vi "Sim Signal 1 CH.vi"(8 "Voltage 2":dbl, 9 "Filter 2":enum16{"Highpass", "Lowpass"}(ring), 10 "Filter 1":enum16{"Highpass", "Lowpass"}(ring), 11 "Voltage 1":dbl) -> (3 "Signal 1 Out":dbl)   [LabVIEW 2010]
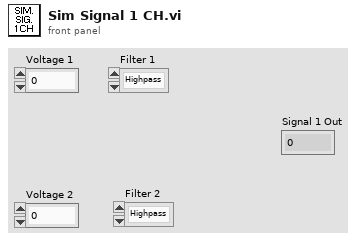
[diagram p1: front panel]
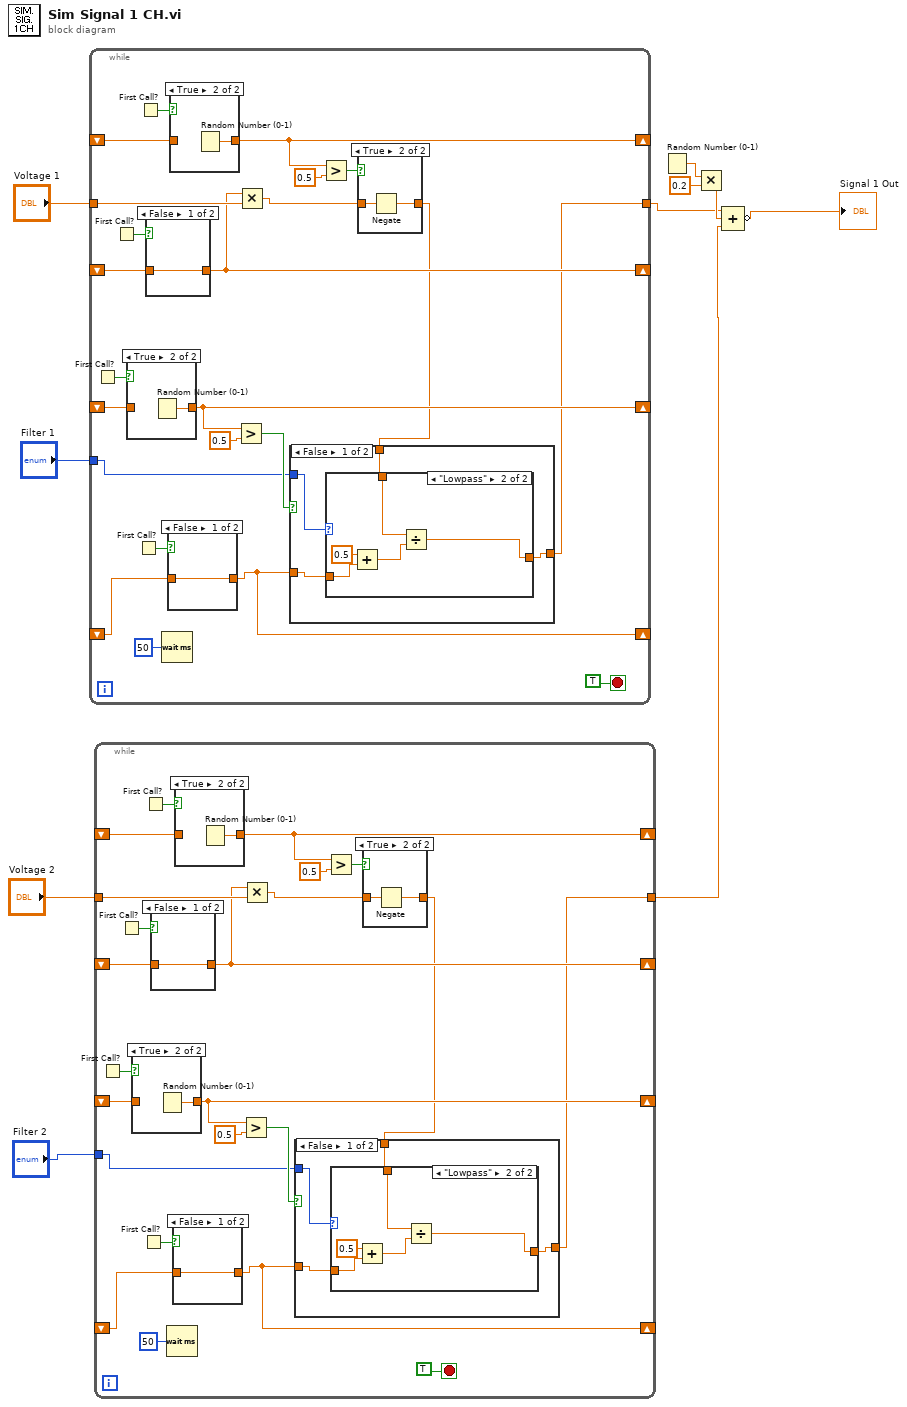
[diagram p0: block diagram]
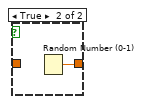
[diagram p2: hidden frame]
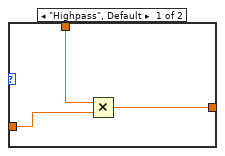
[diagram p3: hidden frame]
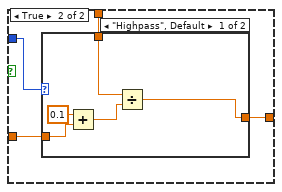
[diagram p4: hidden frame]
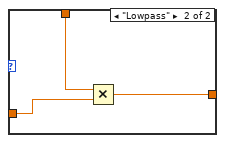
[diagram p5: hidden frame]
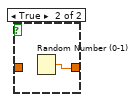
[diagram p9: hidden frame]
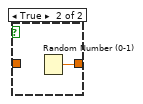
[diagram p10: hidden frame]
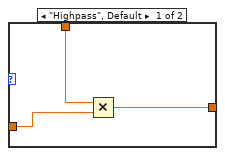
[diagram p11: hidden frame]
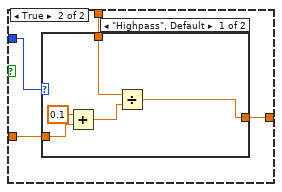
[diagram p12: hidden frame]
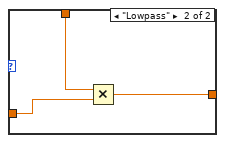
[diagram p13: hidden frame]
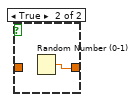
[diagram p17: hidden frame]
diagram:
  n1 = while {
    tunnel: "Voltage 1" -> [w33]
    shift-right: [w31] -> _
    shift-left: _ -> [w30]
    tunnel: [w13] -> w5
    shift-right: [w26] -> _
    shift-left: _ -> [w25]
    tunnel: "Filter 1" -> [w17]
    shift-right: [w20] -> _
    shift-left: _ -> [w19]
    shift-right: [w12] -> _
    shift-left: _ -> [w11]
    stop <- TRUE stop-if-true
    n2 = First Call?() -> (First Call?: T/F=w22:bool)
    n3 = First Call?() -> (First Call?: T/F=w32:bool)
    n4 = case shown="True" w22 {
      tunnel: [w60 w61] -> w20
      tunnel: w19 -> [w60 _]
      frame False {
      }
      frame True {
        n5 = Random Number (0-1)() -> (number: 0 to 1=w61:dbl)
      }
    }
    n6 = First Call?() -> (First Call?: T/F=w14:bool)
    n7 = First Call?() -> (First Call?: T/F=w29:bool)
    n8 = case shown="False" w32 {
      tunnel: [w67 w68] -> w31
      tunnel: w30 -> [w67 _]
      frame False {
      }
      frame True {
        n9 = Random Number (0-1)() -> (number: 0 to 1=w68:dbl)
      }
    }
    n10 = Wait (ms)(milliseconds to wait=u32 50) -> ()  [unwired: 1 out]
    n11 = case shown="False" w14 {
      tunnel: [w34 w35] -> w12
      tunnel: w11 -> [w34 _]
      frame False {
      }
      frame True {
        n12 = Random Number (0-1)() -> (number: 0 to 1=w35:dbl)
      }
    }
    n13 = case shown="True" w29 {
      tunnel: [w65 w66] -> w26
      tunnel: w25 -> [w65 _]
      frame False {
      }
      frame True {
        n14 = Random Number (0-1)() -> (number: 0 to 1=w66:dbl)
      }
    }
    n15 = Greater?(x=w20, y=0.5) -> (0:w18:bool)
    n16 = Multiply(x=w31, y=w33) -> (x*y=w16:dbl)
    n17 = Greater?(x=w26, y=0.5) -> (0:w27:bool)
    n18 = case shown="True" w27 {
      tunnel: w16 -> [w62 w64]
      tunnel: [w62 w63] -> w15
      frame False {
      }
      frame True {
        n19 = Negate(x=w64) -> (-x=w63:dbl)
      }
    }
    n20 = case shown="False" w18 {
      tunnel: w17 -> [w36 w51]
      tunnel: w15 -> [w38 w50]
      tunnel: w12 -> [w39 w49]
      tunnel: [w37 w48] -> w13
      frame False {
        n21 = case shown="\"Lowpass\"" w36 {
          tunnel: w38 -> [w41 w47]
          tunnel: w39 -> [w42 w46]
          tunnel: [w40 w43] -> w37
          frame "Highpass", Default {
            n22 = Multiply(x=w41, y=w42) -> (x*y=w40:dbl)
          }
          frame "Lowpass" {
            n23 = Add(x=0.5, y=w46) -> (x+y=w44:dbl)
            n24 = Divide(x=w47, y=w44) -> (x/y=w43:dbl)
          }
        }
      }
      frame True {
        n25 = case shown="\"Highpass\", Default" w51 {
          tunnel: w50 -> [w56 w58]
          tunnel: w49 -> [w55 w59]
          tunnel: [w52 w57] -> w48
          frame "Highpass", Default {
            n26 = Add(x=0.1, y=w55) -> (x+y=w53:dbl)
            n27 = Divide(x=w56, y=w53) -> (x/y=w52:dbl)
          }
          frame "Lowpass" {
            n28 = Multiply(x=w58, y=w59) -> (x*y=w57:dbl)
          }
        }
      }
    }
  }
  n29 = while {
    tunnel: "Voltage 2" -> [w91]
    shift-right: [w89] -> _
    shift-left: _ -> [w88]
    tunnel: [w71] -> w1
    shift-right: [w84] -> _
    shift-left: _ -> [w83]
    tunnel: "Filter 2" -> [w75]
    shift-right: [w78] -> _
    shift-left: _ -> [w77]
    shift-right: [w70] -> _
    shift-left: _ -> [w69]
    stop <- TRUE stop-if-true
    n30 = First Call?() -> (First Call?: T/F=w80:bool)
    n31 = First Call?() -> (First Call?: T/F=w90:bool)
    n32 = case shown="True" w80 {
      tunnel: [w118 w119] -> w78
      tunnel: w77 -> [w118 _]
      frame False {
      }
      frame True {
        n33 = Random Number (0-1)() -> (number: 0 to 1=w119:dbl)
      }
    }
    n34 = First Call?() -> (First Call?: T/F=w72:bool)
    n35 = First Call?() -> (First Call?: T/F=w87:bool)
    n36 = case shown="False" w90 {
      tunnel: [w125 w126] -> w89
      tunnel: w88 -> [w125 _]
      frame False {
      }
      frame True {
        n37 = Random Number (0-1)() -> (number: 0 to 1=w126:dbl)
      }
    }
    n38 = Wait (ms)(milliseconds to wait=u32 50) -> ()  [unwired: 1 out]
    n39 = case shown="False" w72 {
      tunnel: [w92 w93] -> w70
      tunnel: w69 -> [w92 _]
      frame False {
      }
      frame True {
        n40 = Random Number (0-1)() -> (number: 0 to 1=w93:dbl)
      }
    }
    n41 = case shown="True" w87 {
      tunnel: [w123 w124] -> w84
      tunnel: w83 -> [w123 _]
      frame False {
      }
      frame True {
        n42 = Random Number (0-1)() -> (number: 0 to 1=w124:dbl)
      }
    }
    n43 = Greater?(x=w78, y=0.5) -> (0:w76:bool)
    n44 = Multiply(x=w89, y=w91) -> (x*y=w74:dbl)
    n45 = Greater?(x=w84, y=0.5) -> (0:w85:bool)
    n46 = case shown="True" w85 {
      tunnel: w74 -> [w120 w122]
      tunnel: [w120 w121] -> w73
      frame False {
      }
      frame True {
        n47 = Negate(x=w122) -> (-x=w121:dbl)
      }
    }
    n48 = case shown="False" w76 {
      tunnel: w75 -> [w94 w109]
      tunnel: w73 -> [w96 w108]
      tunnel: w70 -> [w97 w107]
      tunnel: [w95 w106] -> w71
      frame False {
        n49 = case shown="\"Lowpass\"" w94 {
          tunnel: w96 -> [w99 w105]
          tunnel: w97 -> [w100 w104]
          tunnel: [w98 w101] -> w95
          frame "Highpass", Default {
            n50 = Multiply(x=w99, y=w100) -> (x*y=w98:dbl)
          }
          frame "Lowpass" {
            n51 = Add(x=0.5, y=w104) -> (x+y=w102:dbl)
            n52 = Divide(x=w105, y=w102) -> (x/y=w101:dbl)
          }
        }
      }
      frame True {
        n53 = case shown="\"Highpass\", Default" w109 {
          tunnel: w108 -> [w114 w116]
          tunnel: w107 -> [w113 w117]
          tunnel: [w110 w115] -> w106
          frame "Highpass", Default {
            n54 = Add(x=0.1, y=w113) -> (x+y=w111:dbl)
            n55 = Divide(x=w114, y=w111) -> (x/y=w110:dbl)
          }
          frame "Lowpass" {
            n56 = Multiply(x=w116, y=w117) -> (x*y=w115:dbl)
          }
        }
      }
    }
  }
  n57 = Random Number (0-1)() -> (number: 0 to 1=w8:dbl)
  n58 = Multiply(x=w8, y=0.2) -> (x*y=w6:dbl)
  n59 = Compound Arithmetic op=ADD(w5, w6, w1) -> (invert →"Signal 1 Out":dbl)
